vi "Get Method Prototype.vi"(8 "error in (no error)":errorcluster, 10 "Method Name":string, 11 "SMOFacade in":refnum<class "SMOFacade.lvclass">) -> (0 "error out":errorcluster, 2 "Method Prototype":string, 3 "SMOFacade out":refnum<class "SMOFacade.lvclass">, 4 "Default Output":variant, 5 "Default Input":variant)   [LabVIEW 2019, in "SMOFacade.lvclass"]
doc: "JKI State Machine Objects (SMO) 1.3.0.56\nJKI - JKI\nCopyright (c) 2017, JKI"
uses:
  SMOFacade.lvclass
  SMOFacade.lvclass/SMOFacade.ctl
  Registry/SMO_API--Cluster.ctl
  Terminal/Terminal.lvclass
  Registry/Registry-SMO.lvclass
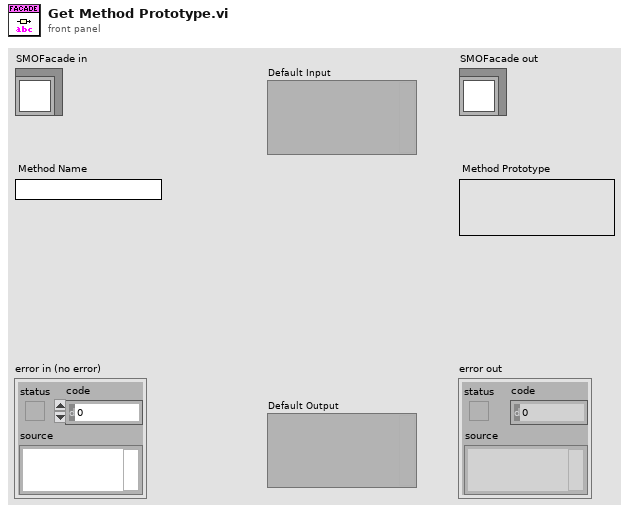
[diagram p1: front panel]
types:
  T1 = typedef "Registry-SMO.lvclass/SMO_API--Cluster.ctl" = cluster{"Method Name":string, "Full Method Name":string, "SMO Input":refnum<class "Terminal.lvclass">, "SMO Output":refnum<class "Terminal.lvclass">, "Inputs":refnum<class "Terminal.lvclass">[], "Outputs":refnum<class "Terminal.lvclass">[], "Error Output":refnum<class "Terminal.lvclass">, "vi reference":refnum<vi>}
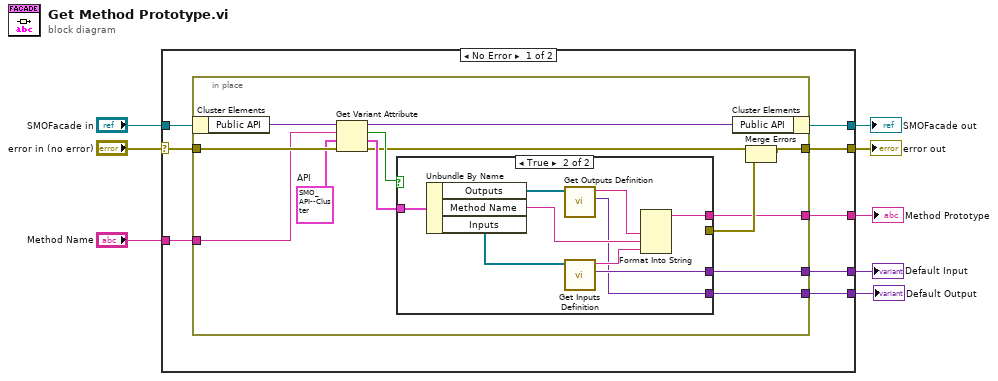
[diagram p0: block diagram]
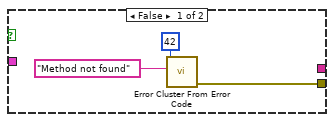
[diagram p2: hidden frame]
diagram:
  n1 = case shown="No Error" "error in (no error)" {
    selector: "error in (no error)" -> [w14 w43]
    tunnel: [w13 w43] -> w7
    tunnel: [w15 w42] -> w5
    tunnel: "SMOFacade in" -> [w16 w42]
    tunnel: "Method Name" -> [w12 _]
    tunnel: [w11 _] -> w3
    tunnel: [w10 _] -> w2
    tunnel: [w9 _] -> w1
    frame No Error {
      n2 = in-place {
        in-place-border: w14 -> [w27]
        in-place-border: [w22] -> w13
        in-place-border: w12 -> [w26]
        in-place-border: [w19] -> w11
        in-place-border: [w18] -> w10
        in-place-border: [w17] -> w9
        w25 = T1 {"Method Name"="", "Full Method Name"="", "SMO Input"=refnum, "SMO Output"=refnum, "Inputs"=[], "Outputs"=[], "Error Output"=refnum, "vi reference"=refnum}  # API
        n3 = in-place-cluster #1(w16) -> ("Public API"=w29:variant)
        n4 = Get Variant Attribute(Variant=w29, name=w26, default value (empty Variant)=w25, error in=w27) -> (duplicate Variant=w28:variant, found=w24:bool, value=w23:T1, error out=w21:errorcluster)
        n5 = case shown="True" w24 {
          tunnel: w23 -> [_ w41]
          tunnel: [w32 _] -> w20
          tunnel: [_ w35] -> w19
          tunnel: [_ w34] -> w18
          tunnel: [_ w33] -> w17
          frame False {
            n6 = call <vilib>:"Error Cluster From Error Code.vi"("error message (\"\")"="Method not found" ("error message (\"\")"), "error code (0)"=42) -> ("error out"=w32:errorcluster)  [unwired: 7 in]
          }
          frame True {
            n7 = Unbundle By Name(w41) -> ("Outputs"=w39:refnum<class "Terminal.lvclass">[], "Method Name"=w37:string, "Inputs"=w40:refnum<class "Terminal.lvclass">[])
            n8 = call "Get Outputs Definition.vi"("Outputs"=w39) -> ("Default Output"=w33:variant, "output string"=w38:string)  [unwired: 9 in]
            n9 = call "Get Inputs Definition.vi"("Inputs"=w40) -> ("Default Input"=w34:variant, "input string"=w36:string)  [unwired: 9 in]
            n10 = Format Into String(w38, w37, w36) -> (resulting string=w35:string)  [unwired: 3 in, 1 out]
          }
        }
        n11 = in-place-cluster #1("Public API"=w28) -> (w15:refnum<class "SMOFacade.lvclass">)
        n12 = Merge Errors(w21, w20) -> (w22:errorcluster)
      }
    }
    frame Error {
    }
  }
  "error out" <- w7
  "SMOFacade out" <- w5
  "Method Prototype" <- w3
  "Default Input" <- w2
  "Default Output" <- w1
